vi "TCP-Send Command.vi"(0 "PXI Address":string, 5 "Port":i32, 7 "Command":string, 9 "timeout (ms)":i32=5000, 11 "error in (no error)":errorcluster, 12 "fast response":bool, 13 "byte order":T1(ring)=enum."native, host order") -> (15 "error out":errorcluster)   [LabVIEW 2020]
panel:
  out "result":i32
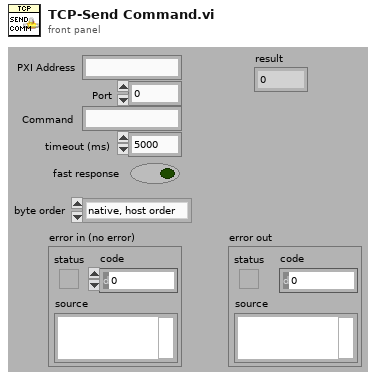
[diagram p1: front panel]
types:
  T1 = enum16{"big-endian, network order", "native, host order", "little-endian"}
  T2 = enum16{"Standard", "Buffered", "CRLF", "Immediate"}
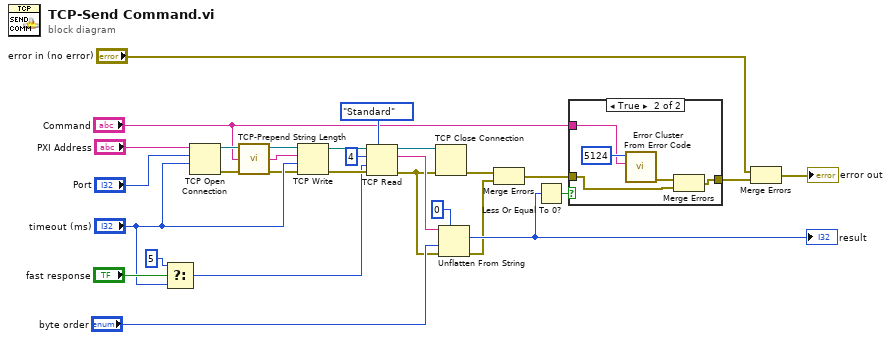
[diagram p0: block diagram]
diagram:
  n1 = Select(t=5 ("timeout ms (25000)"), s="fast response", f="timeout (ms)") -> (s? t:f=w12:i32)
  n2 = TCP Open Connection(address="PXI Address", remote port or service name="Port", timeout ms (60000)="timeout (ms)") -> (connection ID=w25:refnum<k5>, error out=w10:errorcluster)  [unwired: 2 in]
  n3 = call "TCP-Prepend String Length.vi"("Command"="Command") -> ("String"=w8:string)  [unwired: 4 in]
  n4 = TCP Write(connection ID=w25, data in=w8, error in (no error)=w10, 9:"timeout (ms)") -> (connection ID out=w24:refnum<k5>, error out=w15:errorcluster)  [unwired: 1 out]
  n5 = TCP Read(connection ID=w24, bytes to read=4, error in (no error)=w15, 7:T2."Standard" ("mode (standard)"), 9:w12) -> (connection ID out=w23:refnum<k5>, data out=w7:string, error out=w3:errorcluster)
  n6 = TCP Close Connection(connection ID=w23, error in (no error)=w3) -> (error out=w17:errorcluster)  [unwired: 1 in, 1 out]
  n7 = Unflatten From String(type=0, binary string=w7, byte order (0:big-endian, network order)="byte order", error in (no error)=w3) -> (value=w4:i32, error out=w1:errorcluster)  [unwired: 1 in, 1 out]
  "result" <- w4
  n8 = Merge Errors(w17, w1) -> (w2:errorcluster)
  n9 = Less Or Equal To 0?(x=w4) -> (x <= 0?=w22:bool)
  n10 = case shown="True" w22 {
    tunnel: [w28 w30] -> w21
    tunnel: w2 -> [w28 w29]
    tunnel: "Command" -> [_ w31]
    frame False {
    }
    frame True {
      n11 = call <vilib>:"Error Cluster From Error Code.vi"("error message (\"\")"=w31, "error code (0)"=5124) -> ("error out"=w33:errorcluster)  [unwired: 7 in]
      n12 = Merge Errors(w33, w29) -> (w30:errorcluster)
    }
  }
  n13 = Merge Errors("error in (no error)", w21) -> (→"error out":errorcluster)
